vi "readTestDescription.vi"(8 "error in (no error)":errorcluster, 11 "Prueba01 in":refnum<class "Prueba01.lvclass">) -> (0 "error out":errorcluster, 2 "Test Description":string, 3 "Prueba01 out":refnum<class "Prueba01.lvclass">)   [LabVIEW 2019]
uses:
  Prueba01.lvclass
  D:/Users/Patricio/Documents/procal-achs/Pruebas/Prueba/Prueba.lvclass
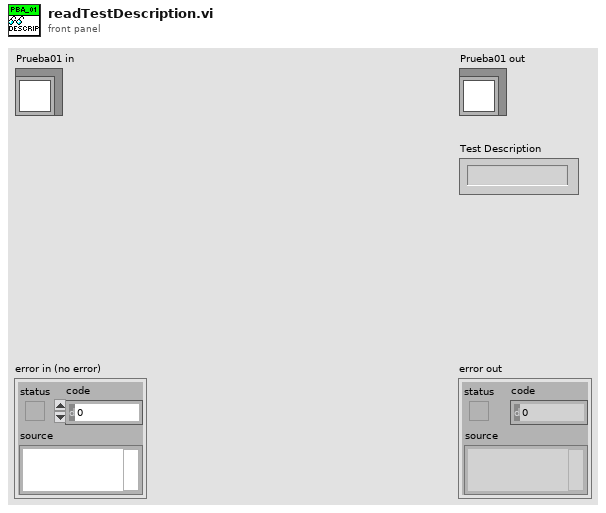
[diagram p1: front panel]
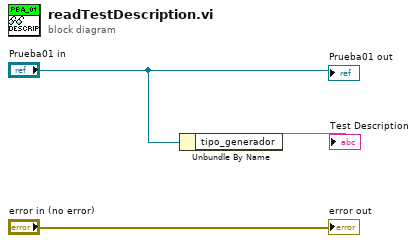
[diagram p0: block diagram]
diagram:
  n1 = Unbundle By Name("Prueba01 in") -> ("tipo_generador"=→"Test Description")
  "error out" <- "error in (no error)"
  "Prueba01 out" <- "Prueba01 in"
